vi "Write to 3.vi"(11 "Test Case In":refnum<class "Tests Event MessengerM.lvclass">) -> (0 "error out":errorcluster, 3 "Test Case Out":refnum<class "Tests Event MessengerM.lvclass">)   [LabVIEW 2020, in "Tests Event MessengerM.lvclass"]
uses:
  Tests Event MessengerM.lvclass
  Tests Event MessengerM.lvclass/Tests Event MessengerM.ctl
  <vilib>/Astemes/LUnit/Test Case.lvclass
  d5a096de-ecbb-44ca-88ac-cb0a84f64389.vi
  4d336554-fddb-4bf2-b660-d711fbeda30d.vi
  01117a10-eca7-47f6-8f47-dfdaea531142.vi
  7df01ec7-e211-4e32-8f06-0271cd9cdc5a.vi
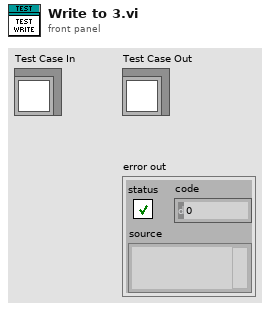
[diagram p1: front panel]
types:
  T1 = typedef "Event MessengerM-c(str,var).lvlib/))Channel.ctl" = refnum<queue>
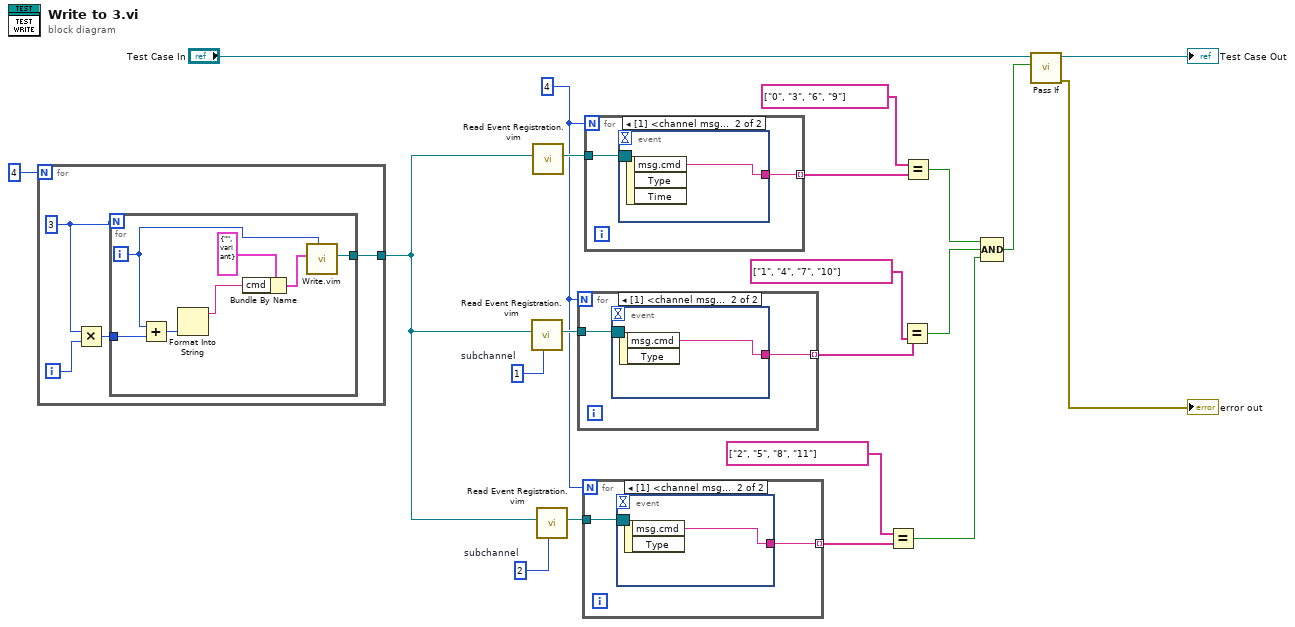
[diagram p0: block diagram]
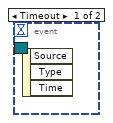
[diagram p2: hidden frame]
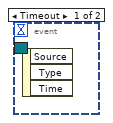
[diagram p3: hidden frame]
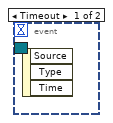
[diagram p4: hidden frame]
diagram:
  w1 = 2  # subchannel
  w8 = 4
  w2 = 1  # subchannel
  n1 = for {
    N: 4 -> [_]
    tunnel: [w25] -> w3
    i -> [w24]
    w22 = 3
    n2 = Multiply(x=w22, y=w24) -> (x*y=w23:i32)
    n3 = for {
      N: w22 -> [_]
      tunnel: [w29] -> w25
      tunnel: w23 -> [w28]
      i -> [w26]
      n4 = Add(x=w26, y=w28) -> (x+y=w27:i32)
      n5 = Format Into String(w27) -> (resulting string=w31:string)  [unwired: 3 in, 1 out]
      n6 = Bundle By Name(cluster=cluster{"cmd":string, "data":variant} {"cmd"="", "data"=variant} ("element"), "cmd"=w31) -> (w30:cluster{"cmd":string, "data":variant})
      n7 = call "Write.vim"("subchannel"=w26, "element"=w30) -> ("channel"=w29:T1)  [unwired: 8 in, 1 out]
    }
  }
  n8 = call "Read Event Registration.vim"("subchannel"=w2, "channel"=w3) -> ("event registration refnum"=w10:refnum<event-registration>)  [unwired: 9 in]
  n9 = call "Read Event Registration.vim"("channel"=w3) -> ("event registration refnum"=w11:refnum<event-registration>)  [unwired: 10 in]
  n10 = call "Read Event Registration.vim"("subchannel"=w1, "channel"=w3) -> ("event registration refnum"=w9:refnum<event-registration>)  [unwired: 9 in]
  n11 = for {
    N: w8 -> [_]
    tunnel: w10 -> [w34]
    tunnel: [w33] -> w18 mode=indexing
    n12 = event shown="[1] <channel msg>: User Event" {
      selector: w34 -> [_ _]
      dyn-events: _ -> [_ _]
      timeout: _ -> [_ _]
      tunnel: [_ w35] -> w33
      event Timeout {
        n13 = event-data() -> ()  [unwired: 1 in, 3 out]
      }
      event User Event {
        n14 = event-data() -> ("msg.cmd"=w35:string)  [unwired: 1 in, 1 out]
      }
    }
  }
  n15 = for {
    N: w8 -> [_]
    tunnel: w9 -> [w37]
    tunnel: [w36] -> w5 mode=indexing
    n16 = event shown="[1] <channel msg>: User Event" {
      selector: w37 -> [_ _]
      dyn-events: _ -> [_ _]
      timeout: _ -> [_ _]
      tunnel: [_ w38] -> w36
      event Timeout {
        n17 = event-data() -> ()  [unwired: 1 in, 3 out]
      }
      event User Event {
        n18 = event-data() -> ("msg.cmd"=w38:string)  [unwired: 1 in, 1 out]
      }
    }
  }
  n19 = for {
    N: w8 -> [_]
    tunnel: w11 -> [w40]
    tunnel: [w39] -> w15 mode=indexing
    n20 = event shown="[1] <channel msg>: User Event" {
      selector: w40 -> [_ _]
      dyn-events: _ -> [_ _]
      timeout: _ -> [_ _]
      tunnel: [_ w41] -> w39
      event Timeout {
        n21 = event-data() -> ()  [unwired: 1 in, 3 out]
      }
      event User Event {
        n22 = event-data() -> ("msg.cmd"=w41:string)  [unwired: 1 in, 2 out]
      }
    }
  }
  n23 = Equal?(x=string[] ["2", "5", "8", "11"] ("Array 2"), y=w5) -> (x = y?=w4:bool)
  n24 = Equal?(x=w18, y=string[] ["1", "4", "7", "10"] ("Array 2")) -> (x = y?=w16:bool)
  n25 = Equal?(x=string[] ["0", "3", "6", "9"] ("Array"), y=w15) -> (x = y?=w13:bool)
  n26 = Compound Arithmetic op=AND(w13, w16, w4) -> (w12:bool)
  n27 = call <vilib>:"Pass If.vi"("Pass?"=w12, "LUnit Test Case In"="Test Case In") -> ("error out"=→"error out":errorcluster, "LUnit Test Case Out"=→"Test Case Out":refnum<class "Tests Event MessengerM.lvclass">)  [unwired: 8 in]
